vi "run_old.vi"(8 "error in (no error)":errorcluster, 11 "DL090409StageScaffold in":refnum<class "StageDL090409Scaffold.lvclass">) -> (0 "error out":errorcluster, 3 "DL090409StageScaffold out":refnum<class "StageDL090409Scaffold.lvclass">)   [LabVIEW 2010]
uses:
  StageDL090409Scaffold.lvsc/Inputs.ctl
  StageDL090409Scaffold.lvsc
  StageDL090409Scaffold.lvsc/Outputs.ctl
  StageDL090409Scaffold.lvsc/Trigger.ctl
  <vilib>/Statechart/Infrastructure/RTStatechart/RunTime SCN.xnode
  StageDL090409Scaffold.lvsc/State.ctl
  StageDL090409Scaffold.lvsc/StatechartState.ctl
  GenericStage/GenericStage/GenericStage.lvclass
  common/classes/SpaceVector/SpaceVector/SpaceVector.lvclass
  GenericStage/GenericStage/translation_mode_enum.ctl
  Display/GenericDisplay/GenericDisplay/GenericDisplay.lvclass
  common/classes/Image/Image/Image.lvclass
  stored_data_cluster.ctl
  StageDL090409Scaffold.lvclass
  GenericStage/GenericStage/trigger_enum.ctl
  common/classes/ErrorController/ErrorController/ErrorController.lvclass
  <vilib>/Statechart/Common/IntGuid.ctl
  <vilib>/Statechart/Common/NI_SC_LVSCCommonFiles.lvlib
  StageDL090409Scaffold.lvsc/CompanionDiagram.vi/15/SC Main.vi
  <vilib>/Statechart/Common/DbgID.ctl
  common/classes/GenericComponent/GenericComponent/GenericComponent.lvclass
panel:
  in  "button:undock":bool
  in  "Tab Control":enum32{"User", "Debug", "About"}(tab)
  out "current x":dbl[unit] caption="x"
  out "current y":dbl[unit] caption="y"
  out "current z":dbl[unit] caption="z"
  in  "setOriginButton":bool
  in  "step x":dbl[unit] caption="x"
  in  "step y":dbl[unit] caption="y"
  in  "step z":dbl[unit] caption="z"
  in  "stepButton":bool
  in  "returnToOriginButton":bool
  in  "Stored positions":i32(listbox)
  in  "Description":string
  in  "store button":bool
  out "position image":T1(plugin-control)
  in  "go to stored button":bool
  in  "remove stored item":bool
  out "active states":T2=[enum."NI.SC.Initial"]
  out "statechart error":errorcluster
  out "statechart loop counter":i32
  out "last trigger":T4
  out "finished?":bool
  # "Move"
  # "Current position"
  # "StageDL090409Scaffold (or child class)\n\nimplemented by: Dominik Langer, University of Zurich\nmodified by: Marcel van 't Hoff, University of Zurich"
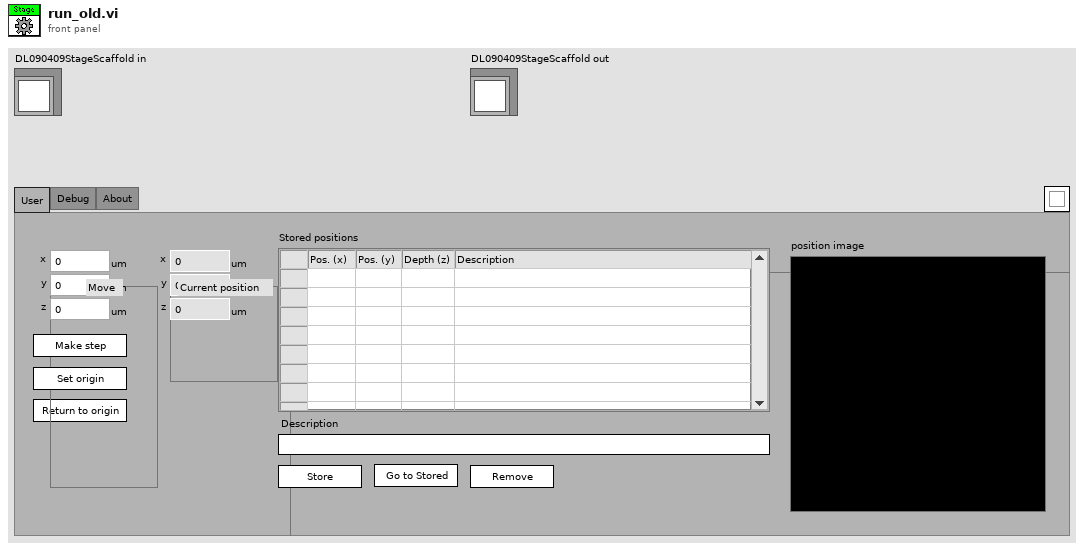
[diagram p1: front panel]
types:
  T1 = typedef "IMAQ Image.ctl" = refnum<image>
  T2 = typedef "StageDL090409Scaffold.lvsc/StatechartState.ctl" = T3[]
  T3 = typedef "StageDL090409Scaffold.lvsc/State.ctl" = enum16{"NI.SC.Initial", "NI.SC.History", "NI.SC.ShallowHistory", "NI.SC.Terminal", "terminating", "running", "initialising", "running\\NI.SC.UnnamedRegion 0\\setting origin", "running\\NI.SC.UnnamedRegion 0\\updating position", "running\\NI.SC.UnnamedRegion 0\\moving", "running\\NI.SC.UnnamedRegion 0\\idle"}
  T4 = typedef "StageDL090409Scaffold.lvsc/Trigger.ctl" = enum16{"NULL", "initialise", "terminate", "move", "update position", "set origin", "return to origin"}
  T5 = typedef "StageDL090409Scaffold.lvsc/Inputs.ctl" = cluster{"error":errorcluster}
  T6 = typedef "NI_SC_LVSCCommonFiles.lvlib/IntGuid.ctl" = cluster{"Data1":u32, "Data2":u16, "Data3":u16, "Data4":u8, "Data5":u8, "Data6":u8, "Data11":u8, "Data9":u8, "Data10":u8, "Data8":u8, "Data7":u8}
  T7 = typedef "NI_SC_LVSCCommonFiles.lvlib/DbgID.ctl" = cluster{"VIRef":u32, "IntGUID":T6}
  T8 = typedef "GenericStage.lvclass/trigger_enum.ctl" = enum16{"NULL", "move", "update position", "set origin", "return to origin"}
  T9 = typedef "GenericStage.lvclass/translation_mode_enum.ctl" = enum16{"DON'T MOVE", "relative", "absolute"}
  T10 = typedef "StageDL090409Scaffold.lvclass/stored_data_cluster.ctl" = cluster{"stored position":refnum<class "SpaceVector.lvclass">, "description":string, "position image":refnum<class "Image.lvclass">}
  T11 = typedef "StageDL090409Scaffold.lvclass/internal_trigger_enum.ctl" = enum16{"NULL", "initialise", "terminate", "move", "update position", "set origin", "return to origin", "attach observer", "detach observer"}
  T12 = typedef "StageDL090409Scaffold.lvsc/Outputs.ctl" = cluster{"error":errorcluster}
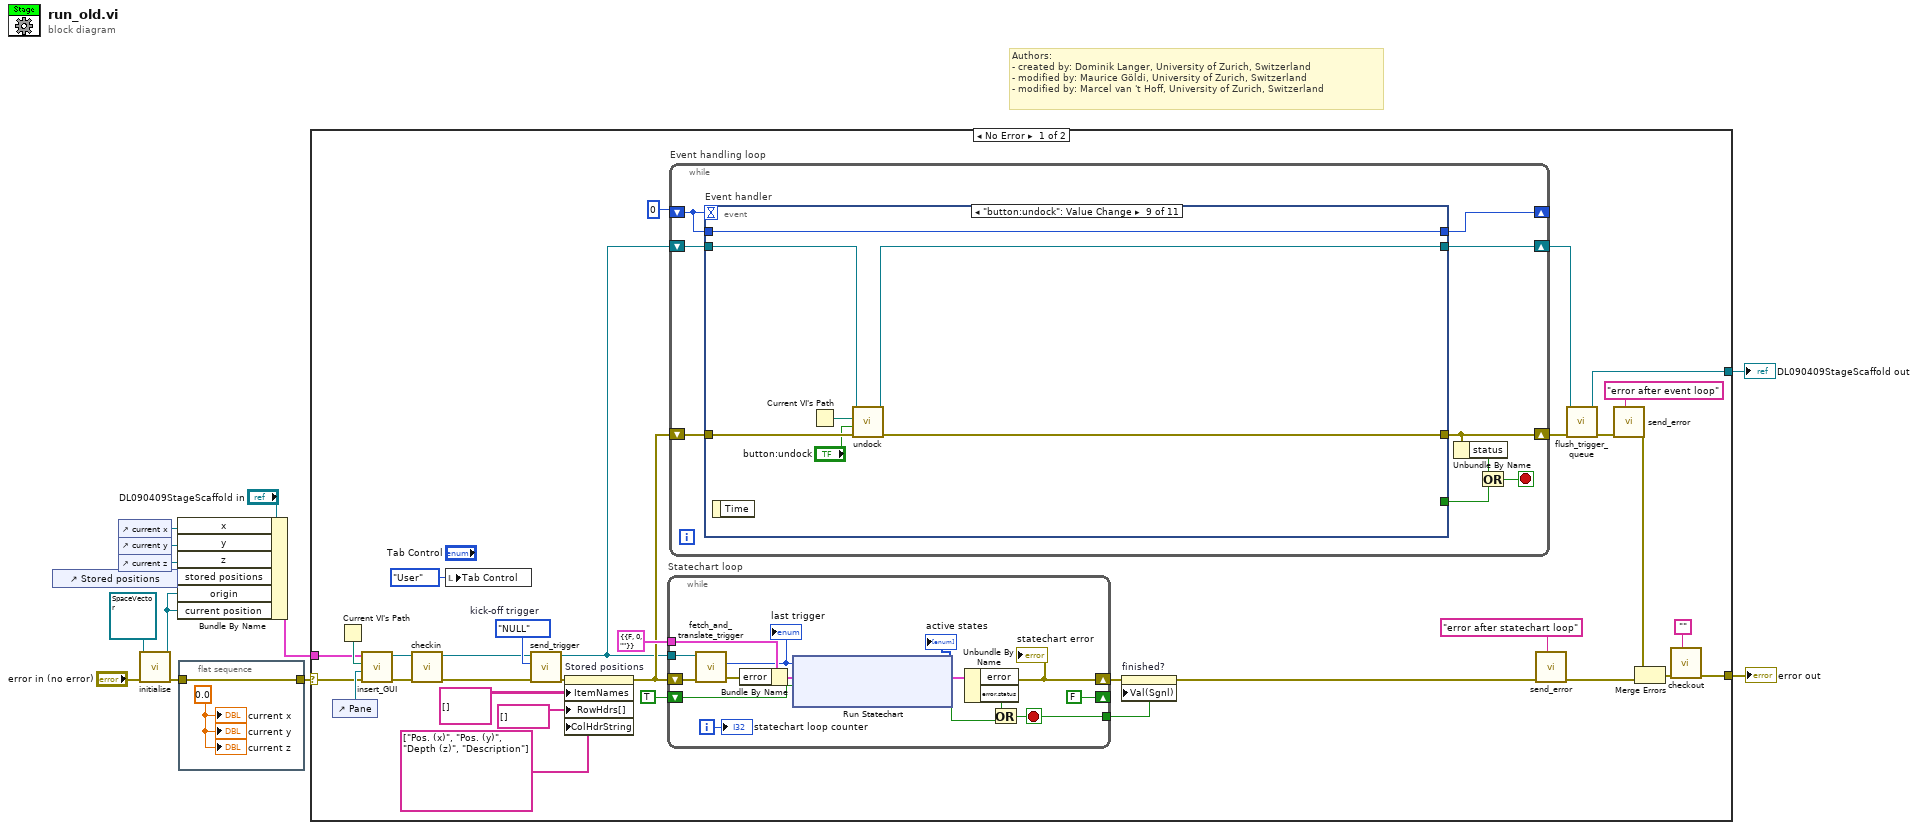
[diagram p0: block diagram]
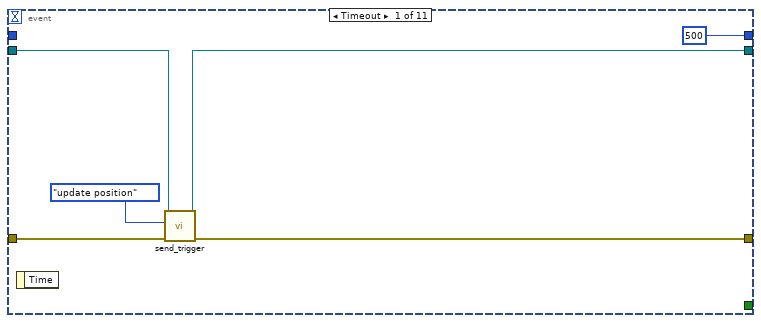
[diagram p2: hidden frame]
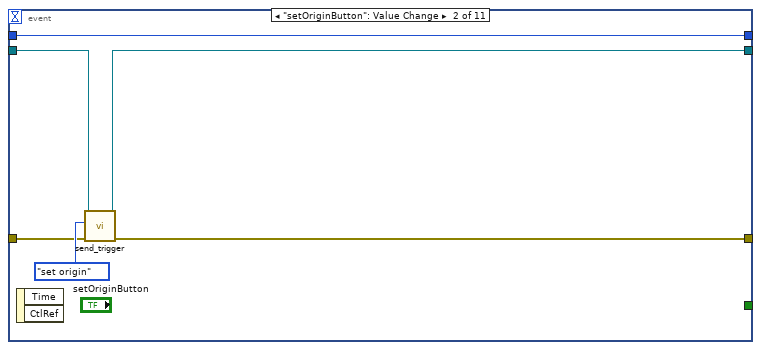
[diagram p3: hidden frame]
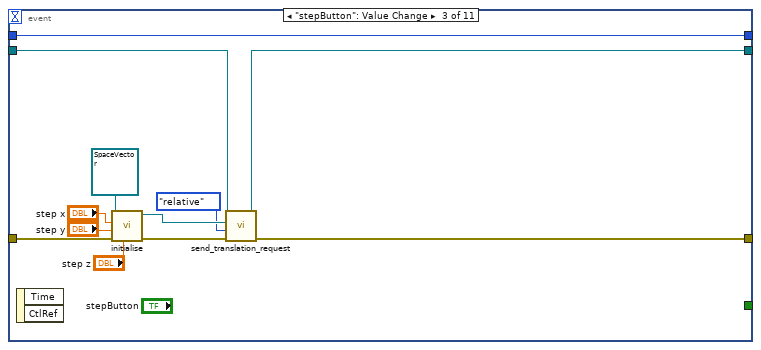
[diagram p4: hidden frame]
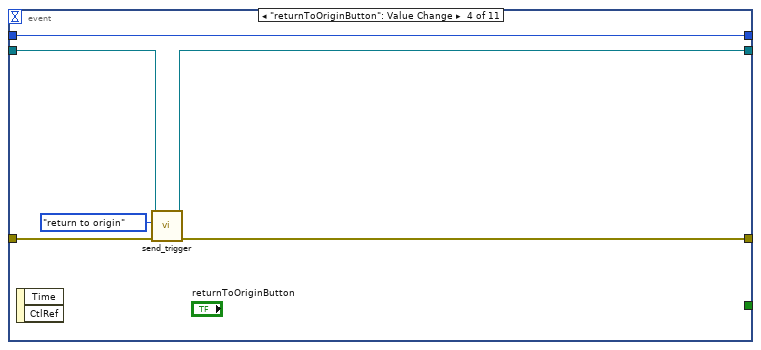
[diagram p5: hidden frame]
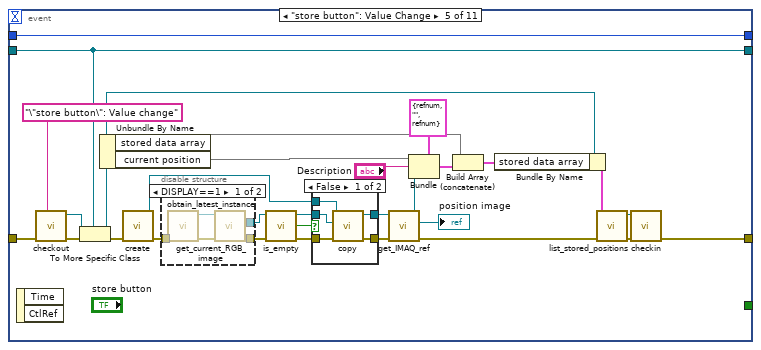
[diagram p6: hidden frame]
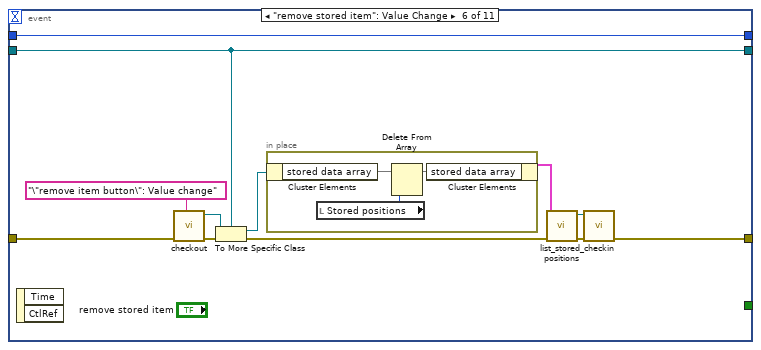
[diagram p9: hidden frame]
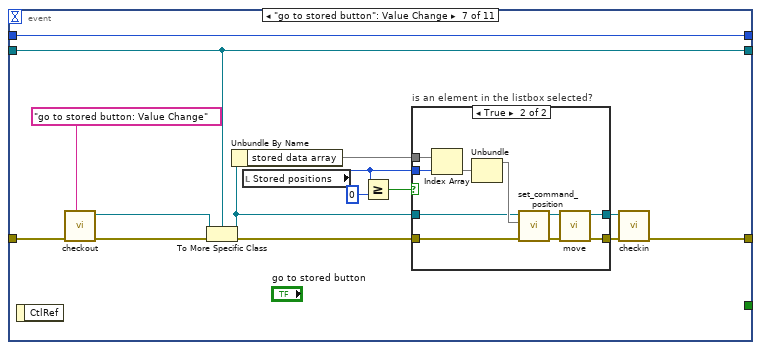
[diagram p10: hidden frame]
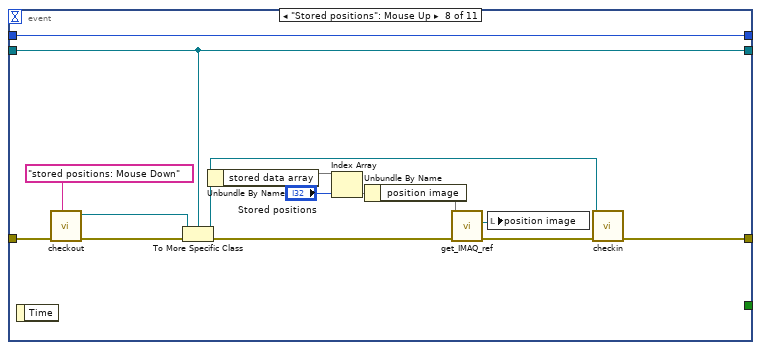
[diagram p12: hidden frame]
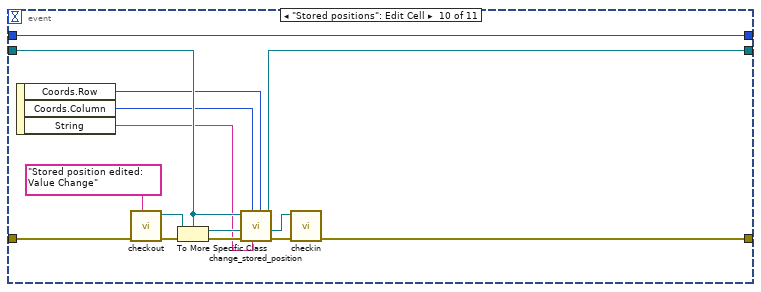
[diagram p13: hidden frame]
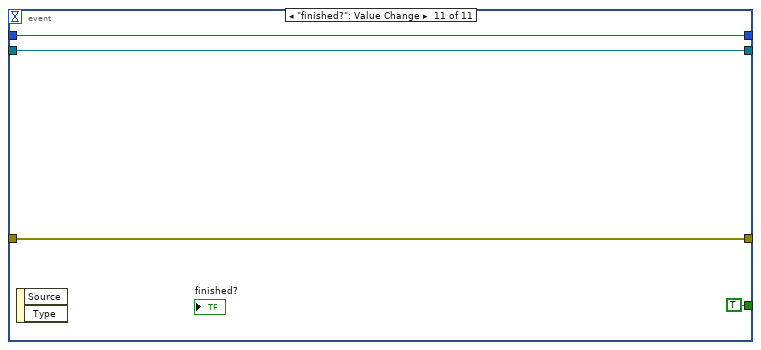
[diagram p14: hidden frame]
diagram:
  # "Authors: \n- created by: Dominik Langer, University of Zurich, Switzerland\n- modified by: Maurice Göldi, University of Zurich, Switzerland\n- modified by: Marcel van 't Hoff, University of Zurich, Switzerland"
  n1 = control-ref of="Stored positions"() -> (w6:refnum<vi>)
  n2 = control-ref of="current x"() -> (w9:refnum<vi>)
  n3 = control-ref of="current y"() -> (w8:refnum<vi>)
  n4 = control-ref of="current z"() -> (w7:refnum<vi>)
  n5 = call "initialise.vi"("error in (no error)"="error in (no error)", "SpaceVector in"=refnum<class "SpaceVector.lvclass"> refnum ("current position")) -> ("error out"=w2:errorcluster, "SpaceVector out"=w4:refnum<class "SpaceVector.lvclass">)  [unwired: 3 in, 5 out]
  n6 = Bundle By Name(cluster="DL090409StageScaffold in", "x"=w9, "y"=w8, "z"=w7, "stored positions"=w6, "origin"=w4, "current position"=w4) -> (w10:cluster{})
  n7 = flat-sequence {
    tunnel: w2 -> [w14]
    tunnel: [w14] -> w1
    frame #0 {
      w15 = dbl[unit] 0.0 ("current x")
      "current x" <- w15
      "current y" <- w15
      "current z" <- w15
    }
  }
  n8 = case shown="No Error" w1 {
    selector: w1 -> [w34 w300]
    tunnel: [w46 w300] -> w13
    tunnel: [w16 w299] -> w12
    tunnel: w10 -> [w40 w299]
    frame No Error {
      w30 = trigger_enum."NULL"  # kick-off trigger
      n9 = control-ref of="Pane"() -> (w38:refnum<vi>)
      n10 = Current VI's Path() -> (path=w41:path)
      n11 = call-dynamic "insert_GUI.vi"("error in (no error)"=w34, "Pane"=w38, "VI path"=w41, "GenericComponent in"=w40) -> ("error out"=w26:errorcluster, "GenericComponent out"=w29:refnum<class "GenericComponent.lvclass">)  [unwired: 6 in]
      n12 = call-dynamic "checkin.vi"("error in (no error)"=w26, "GenericStage in"=w29) -> ("error out"=w23:errorcluster, "GenericStage out"=w22:refnum<class "StageDL090409Scaffold.lvclass">)  [unwired: 8 in]
      n13 = local write "Tab Control"(enum32{"User", "Debug", "About"}."User" ("Tab Control")) -> ()
      n14 = call-dynamic "send_trigger.vi"("error in (no error)"=w23, "trigger"=w30, "GenericStage in"=w22) -> ("error out"=w31:errorcluster, "GenericStage out"=w25:refnum<class "StageDL090409Scaffold.lvclass">)  [unwired: 7 in]
      n15 = property on="Stored positions" class="MCListbox (strict)"(error in=w31, "ItemNames"=string[][] [] ("Item Names"), "RowHdrs[]"=string[] [] ("Row Header Strings[]"), "ColHdrString"=string[] ["Pos. (x)", "Pos. (y)", "Depth (z)", "Description"] ("Row Header Strings[]")) -> (error out=w35:errorcluster)  [unwired: 1 in, 1 out]
      n16 = while "Statechart loop" {
        shift-right: [w58] -> w44
        shift-left: w35 -> [w52]
        tunnel: T5 {"error"={"status"=FALSE, "code"=0, "source"=""}} ("Inputs") -> [w60]
        tunnel: [w55] -> w43
        shift-right: [FALSE] -> _
        shift-left: TRUE -> [w54]
        tunnel: w25 -> [w51]
        i -> [w59]
        stop <- w55 stop-if-true
        n17 = call-dynamic "fetch_and_translate_trigger.vi"("error in (no error)"=w52, "StageDL090409Scaffold in"=w51) -> ("error out"=w50:errorcluster, "statechart trigger"=w49:T11)  [unwired: 6 in, 2 out]
        "last trigger" <- w49
        n18 = Bundle By Name(cluster=w60, "error"=w50) -> (w63:T5)
        n19 = xnode "Run Statechart"("Init?"=w54, "Inputs"=w63, "Trigger"=w49) -> ("Terminated?"=w57:bool, "Outputs"=w62:T12, "Active States"=→"active states":T2)
        n20 = Unbundle By Name(w62) -> ("error"=w58:errorcluster, "error.status"=w56:bool)
        "statechart error" <- w58
        n21 = Or(x=w56, y=w57) -> (x .or. y?=w55:bool)
        "statechart loop counter" <- w59
      }
      n22 = while "Event handling loop" {
        shift-right: [w141] -> _
        shift-left: 0 -> [w142]
        shift-right: [w137] -> w18
        shift-left: w35 -> [w140]
        shift-right: [w138] -> w19
        shift-left: w25 -> [w139]
        stop <- w134 stop-if-true
        n23 = event "Event handler" shown="[8] \"button:undock\": Value Change" {
          selector: _ -> [_ _ _ _ _ _ _ _ _ _ _]
          dyn-events: _ -> [_ _ _ _ _ _ _ _ _ _ _]
          timeout: w142 -> [_ _ _ _ _ _ _ _ _ _ _]
          tunnel: w142 -> [_ w154 w166 w172 w202 w227 w245 w272 w279 w294 w298]
          tunnel: [500 w154 w166 w172 w202 w227 w245 w272 w279 w294 w298] -> w141
          tunnel: w140 -> [w144 w149 w165 w168 w201 w222 w240 w265 w278 w293 w297]
          tunnel: [w143 w153 w159 w167 w177 w221 w236 w259 w277 w289 w297] -> w137
          tunnel: [_ _ _ _ _ _ _ _ _ _ TRUE] -> w135
          tunnel: w139 -> [w146 w152 w158 w170 w198 w226 w234 w261 w276 w284 w295]
          tunnel: [w145 w151 w156 w169 w198 w226 w234 w261 w275 w283 w295] -> w138
          event Timeout {
            n24 = event-data() -> ()  [unwired: 2 out]
            n25 = call-dynamic "send_trigger.vi"("error in (no error)"=w144, "trigger"=trigger_enum."update position", "GenericStage in"=w146) -> ("error out"=w143:errorcluster, "GenericStage out"=w145:refnum<class "StageDL090409Scaffold.lvclass">)  [unwired: 7 in]
          }
          event "setOriginButton": Value Change {
            n26 = event-data() -> ()  [unwired: 3 out]
            n27 = call-dynamic "send_trigger.vi"("error in (no error)"=w149, "trigger"=trigger_enum."set origin", "GenericStage in"=w152) -> ("error out"=w153:errorcluster, "GenericStage out"=w151:refnum<class "StageDL090409Scaffold.lvclass">)  [unwired: 7 in]
          }
          event "stepButton": Value Change {
            n28 = event-data() -> ()  [unwired: 3 out]
            n29 = call "initialise.vi"("z"="step z", "error in (no error)"=w165, "y"="step y", "x"="step x", "SpaceVector in"=refnum<class "SpaceVector.lvclass"> refnum ("current position")) -> ("error out"=w160:errorcluster, "SpaceVector out"=w161:refnum<class "SpaceVector.lvclass">)  [unwired: 5 in]
            n30 = call-dynamic "send_translation_request.vi"("error in (no error)"=w160, "translation mode"=translation_mode_enum."relative", "translation vector"=w161, "GenericStage in"=w158) -> ("error out"=w159:errorcluster, "GenericStage out"=w156:refnum<class "StageDL090409Scaffold.lvclass">)  [unwired: 6 in]
          }
          event "returnToOriginButton": Value Change {
            n31 = event-data() -> ()  [unwired: 3 out]
            n32 = call-dynamic "send_trigger.vi"("error in (no error)"=w168, "trigger"=trigger_enum."return to origin", "GenericStage in"=w170) -> ("error out"=w167:errorcluster, "GenericStage out"=w169:refnum<class "StageDL090409Scaffold.lvclass">)  [unwired: 7 in]
          }
          event "store button": Value Change {
            n33 = event-data() -> ()  [unwired: 3 out]
            n34 = call "checkout.vi"("locked by?"="\"store button\": Value change", "error in (no error)"=w201) -> ("error out"=w200:errorcluster, "GenericStage out"=w199:refnum<class "GenericStage.lvclass">)  [unwired: 8 in]
            n35 = To More Specific Class(target class=w198, reference=w199, error in=w200) -> (specific class reference=w185:refnum<class "StageDL090409Scaffold.lvclass">, error out=w193:errorcluster)
            n36 = Unbundle By Name(w185) -> ("stored data array"=w187, "current position"=w190)
            n37 = call "create.vi"("error in (no error)"=w193) -> ("error out"=w192:errorcluster, "Image out"=w191:refnum<class "Image.lvclass">)  [unwired: 9 in]
            n38 = disable-structure shown="DISPLAY==1" {
              disable-tunnel: w192 -> [w205 w208]
              disable-tunnel: [w204 w208] -> w182
              disable-tunnel: [w203 _] -> w180
              frame condition #0 {
                n39 = call "obtain_latest_instance.vi"("error in (no error)"=w205) -> ("error out"=w207:errorcluster, "GenericDisplay out"=w206:refnum<class "GenericDisplay.lvclass">)  [unwired: 9 in]
                n40 = call-dynamic "get_current_RGB_image.vi"("error in (no error)"=w207, "GenericDisplay in"=w206) -> ("error out"=w204:errorcluster, "RGB image"=w203:refnum<class "Image.lvclass">)  [unwired: 7 in, 1 out]
              }
              frame condition #1 (active) {
              }
            }
            n41 = call-dynamic "is_empty.vi"("error in (no error)"=w182, "Image in"=w180) -> ("error out"=w181:errorcluster, "emtpy?"=w178:bool, "Image out"=w179:refnum<class "Image.lvclass">)  [unwired: 7 in]
            n42 = case shown="False" w178 {
              tunnel: [w213 w215] -> w197
              tunnel: [w212 w214] -> w195
              tunnel: w191 -> [w211 w214]
              tunnel: w181 -> [w210 w215]
              tunnel: w179 -> [w209 _]
              frame False {
                n43 = call "copy.vi"("error in (no error)"=w210, "image to copy (source)"=w209, "Image in (target)"=w211) -> ("error out"=w213:errorcluster, "Image out"=w212:refnum<class "Image.lvclass">)  [unwired: 7 in]
              }
              frame True {
              }
            }
            n44 = call-dynamic "get_IMAQ_ref.vi"("error in (no error)"=w197, "Image.lvclass in"=w195) -> ("error out"=w176:errorcluster, "Image"=→"position image":T1, "Image.lvclass out"=w188:refnum<class "Image.lvclass">)  [unwired: 5 in, 2 out]
            n45 = Bundle(cluster=T10 {"stored position"=refnum, "description"="", "position image"=refnum} ("stored data"), "stored position"=w190, "description"="Description", "position image"=w188) -> (w186:T10)
            n46 = Build Array (concatenate)(w187, w186) -> (w183:T10[])
            n47 = Bundle By Name(cluster=w185, "stored data array"=w183) -> (w174:cluster{})
            n48 = call-dynamic "list_stored_positions.vi"("error in (no error)"=w176, "StageDL090409Scaffold in"=w174) -> ("error out"=w175:errorcluster, "StageDL090409Scaffold out"=w173:refnum<class "StageDL090409Scaffold.lvclass">)  [unwired: 8 in]
            n49 = call-dynamic "checkin.vi"("error in (no error)"=w175, "GenericStage in"=w173) -> ("error out"=w177:errorcluster)  [unwired: 8 in, 1 out]
          }
          event "remove stored item": Value Change {
            n50 = event-data() -> ()  [unwired: 3 out]
            n51 = call "checkout.vi"("locked by?"="\"remove item button\": Value change", "error in (no error)"=w222) -> ("error out"=w225:errorcluster, "GenericStage out"=w223:refnum<class "GenericStage.lvclass">)  [unwired: 8 in]
            n52 = To More Specific Class(target class=w226, reference=w223, error in=w225) -> (specific class reference=w217:refnum<class "StageDL090409Scaffold.lvclass">, error out=w220:errorcluster)
            n53 = in-place {
              n54 = in-place-cluster #1(w217) -> ("stored data array"=w229)
              n55 = local read "Stored positions"() -> (w230:i32)
              n56 = Delete From Array(array=w229, index=w230) -> (array with subset deleted=w228)  [unwired: 1 in, 1 out]
              n57 = in-place-cluster #1("stored data array"=w228) -> (w216:cluster{})
            }
            n58 = call-dynamic "list_stored_positions.vi"("error in (no error)"=w220, "StageDL090409Scaffold in"=w216) -> ("error out"=w219:errorcluster, "StageDL090409Scaffold out"=w218:refnum<class "StageDL090409Scaffold.lvclass">)  [unwired: 8 in]
            n59 = call-dynamic "checkin.vi"("error in (no error)"=w219, "GenericStage in"=w218) -> ("error out"=w221:errorcluster)  [unwired: 8 in, 1 out]
          }
          event "go to stored button": Value Change {
            n60 = event-data() -> ()  [unwired: 2 out]
            n61 = call "checkout.vi"("locked by?"="go to stored button: Value Change", "error in (no error)"=w240) -> ("error out"=w239:errorcluster, "GenericStage out"=w237:refnum<class "GenericStage.lvclass">)  [unwired: 8 in]
            n62 = To More Specific Class(target class=w234, reference=w237, error in=w239) -> (specific class reference=w233:refnum<class "StageDL090409Scaffold.lvclass">, error out=w238:errorcluster)
            n63 = Unbundle By Name(w233) -> ("stored data array"=w244)
            n64 = local read "Stored positions"() -> (w242:i32)
            n65 = Greater Or Equal?(x=w242, y=0) -> (x >= y?=w243:bool)
            n66 = case "is an element in the listbox selected?" shown="True" w243 {
              tunnel: w244 -> [_ w257]
              tunnel: [w247 w253] -> w235
              tunnel: w238 -> [w247 w251]
              tunnel: w242 -> [_ w250]
              tunnel: w233 -> [w246 w249]
              tunnel: [w246 w248] -> w232
              frame False {
              }
              frame True {
                n67 = Index Array(array=w257, index=w250) -> (element=w256)
                n68 = Unbundle(w256) -> (w255)  [unwired: 2 out]
                n69 = call-dynamic "set_command_position.vi"("error in (no error)"=w251, "command position"=w255, "DL090409StageScaffold.lvclass in"=w249) -> ("error out"=w254:errorcluster, "DL090409StageScaffold.lvclass out"=w252:refnum<class "StageDL090409Scaffold.lvclass">)  [unwired: 7 in]
                n70 = call-dynamic "move.vi"("error in (no error)"=w254, "DL090409StageScaffold in"=w252) -> ("error out"=w253:errorcluster, "DL090409StageScaffold out"=w248:refnum<class "StageDL090409Scaffold.lvclass">)  [unwired: 8 in]
              }
            }
            n71 = call-dynamic "checkin.vi"("error in (no error)"=w235, "GenericStage in"=w232) -> ("error out"=w236:errorcluster)  [unwired: 8 in, 1 out]
          }
          event "Stored positions": Mouse Up {
            n72 = event-data() -> ()  [unwired: 2 out]
            n73 = call "checkout.vi"("locked by?"="stored positions: Mouse Down", "error in (no error)"=w265) -> ("error out"=w266:errorcluster, "GenericStage out"=w262:refnum<class "GenericStage.lvclass">)  [unwired: 8 in]
            n74 = To More Specific Class(target class=w261, reference=w262, error in=w266) -> (specific class reference=w258:refnum<class "StageDL090409Scaffold.lvclass">, error out=w264:errorcluster)
            n75 = Unbundle By Name(w258) -> ("stored data array"=w271)
            n76 = Index Array(array=w271, index="Stored positions") -> (element=w270)
            n77 = Unbundle By Name(w270) -> ("position image"=w269)
            n78 = call-dynamic "get_IMAQ_ref.vi"("error in (no error)"=w264, "Image.lvclass in"=w269) -> ("error out"=w260:errorcluster, "Image"=w268:T1)  [unwired: 5 in, 3 out]
            n79 = local write "position image"(w268) -> ()
            n80 = call-dynamic "checkin.vi"("error in (no error)"=w260, "GenericStage in"=w258) -> ("error out"=w259:errorcluster)  [unwired: 8 in, 1 out]
          }
          event "button:undock": Value Change {
            n81 = event-data() -> ()  [unwired: 2 out]
            n82 = Current VI's Path() -> (path=w273:path)
            n83 = call-dynamic "undock.vi"("error in (no error)"=w278, "undock?"="button:undock", "VI path"=w273, "GenericComponent in"=w276) -> ("error out"=w277:errorcluster, "GenericComponent out"=w275:refnum<class "StageDL090409Scaffold.lvclass">)  [unwired: 6 in]
          }
          event "Stored positions": Edit Cell {
            n84 = event-data() -> ("Coords.Row"=w280:i32, "Coords.Column"=w282:i32, "String"=w281:string)  [unwired: 1 out]
            n85 = call "checkout.vi"("locked by?"="Stored position edited: Value Change", "error in (no error)"=w293) -> ("error out"=w290:errorcluster, "GenericStage out"=w291:refnum<class "GenericStage.lvclass">)  [unwired: 8 in]
            n86 = To More Specific Class(target class=w284, reference=w291, error in=w290) -> (specific class reference=w288:refnum<class "StageDL090409Scaffold.lvclass">, error out=w287:errorcluster)
            n87 = call-dynamic "change_stored_position.vi"("Row"=w280, "String"=w281, "Column"=w282, "error in (no error)"=w287, "specific class reference"=w288, "StageDL090409Scaffold in"=w284) -> ("error out"=w285:errorcluster, "specific class reference out"=w286:refnum<class "StageDL090409Scaffold.lvclass">, "StageDL090409Scaffold out"=w283:refnum<class "StageDL090409Scaffold.lvclass">)  [unwired: 3 in]
            n88 = call-dynamic "checkin.vi"("error in (no error)"=w285, "GenericStage in"=w286) -> ("error out"=w289:errorcluster)  [unwired: 8 in, 1 out]
          }
          event "finished?": Value Change {
            n89 = event-data() -> ()  [unwired: 3 out]
          }
        }
        n90 = Unbundle By Name(w137) -> ("status"=w136:bool)
        n91 = Or(x=w136, y=w135) -> (x .or. y?=w134:bool)
      }
      n92 = property on="finished?" class="Bool (strict)"(error in=w44, "Val(Sgnl)"=w43) -> (error out=w24:errorcluster)  [unwired: 1 in, 1 out]
      n93 = call "send_error.vi"("additional message"="error after statechart loop", "error in (no error)"=w24) -> ("error out"=w32:errorcluster)  [unwired: 9 in]
      n94 = call-dynamic "flush_trigger_queue.vi"("error in (no error)"=w18, "GenericToplevelComponent in"=w19) -> ("error out"=w17:errorcluster, "GenericToplevelComponent out"=w16:refnum<class "StageDL090409Scaffold.lvclass">)  [unwired: 8 in]
      n95 = call "send_error.vi"("additional message"="error after event loop", "error in (no error)"=w17) -> ("error out"=w33:errorcluster)  [unwired: 9 in]
      n96 = Merge Errors(w33, w32) -> (w47:errorcluster)
      n97 = call "checkout.vi"("locked by?"="", "error in (no error)"=w47) -> ("error out"=w46:errorcluster)  [unwired: 8 in, 1 out]
    }
    frame Error {
    }
  }
  "error out" <- w13
  "DL090409StageScaffold out" <- w12
